vi "Get Pin at Target Pout.vi"(8 "error in":errorcluster, 9 "x-axis name":string, 10 "IM_Target Pout Per Tone (dBm)":dbl, 11 "Graph Data":T1) -> (0 "error out":errorcluster, 3 "Pin @ Target Pout":dbl)   [LabVIEW 2023, in "FPT Intermodulation UI.lvlib"]
uses:
  FPT Intermodulation UI.lvlib
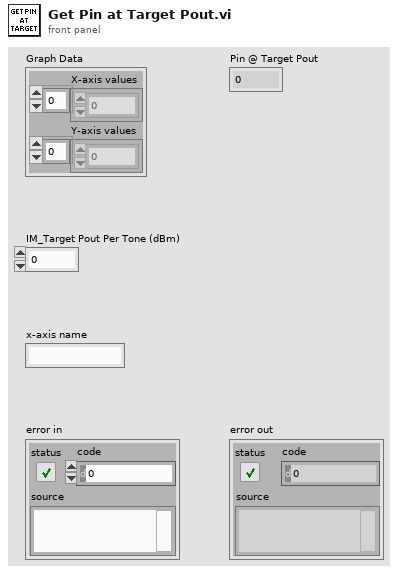
[diagram p1: front panel]
types:
  T1 = cluster{"X-axis values":dbl[], "Y-axis values":dbl[]}
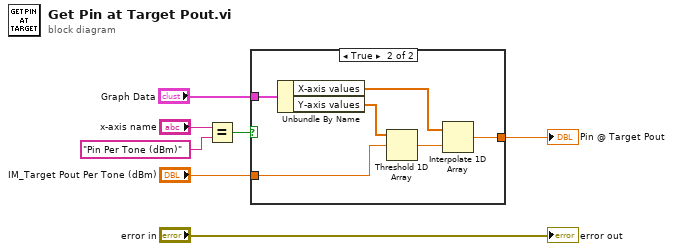
[diagram p0: block diagram]
diagram:
  n1 = Equal?(x="x-axis name", y="Pin Per Tone (dBm)") -> (x = y?=w5:bool)
  n2 = case shown="True" w5 {
    tunnel: "IM_Target Pout Per Tone (dBm)" -> [_ w13]
    tunnel: [_ w11] -> w4
    tunnel: "Graph Data" -> [_ w10]
    frame False {
    }
    frame True {
      n3 = Unbundle By Name(w10) -> ("X-axis values"=w9:dbl[], "Y-axis values"=w8:dbl[])
      n4 = Threshold 1D Array(2:w13, 3:w8) -> (0:w12:dbl)  [unwired: 1 in]
      n5 = Interpolate 1D Array(1:w12, 2:w9) -> (0:w11:dbl)
    }
  }
  "Pin @ Target Pout" <- w4
  "error out" <- "error in"
